vi "RunAClone.vi"(11 "VI in":refnum<vi>) -> (3 "reference out":refnum<vi>)   [LabVIEW 2021]
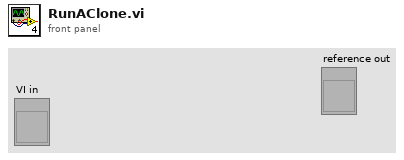
[diagram p1: front panel]
types:
  T1 = enum32{"Invalid", "Standard", "Closed", "Hidden", "Minimized", "Maximized"}
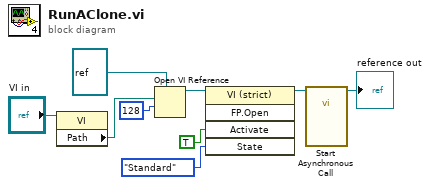
[diagram p0: block diagram]
diagram:
  n1 = property class="VI"(reference="VI in") -> ("Path"=w3:path)  [unwired: 1 in, 2 out]
  n2 = Open VI Reference(type specifier VI Refnum (for type only)=refnum<vi> refnum, vi path=w3, options=128) -> (vi reference=w8:refnum<vi>)  [unwired: 3 in, 1 out]
  n3 = invoke class="VI (strict)" method="FP.Open"(reference=w8, "Activate"=TRUE ("Activate?"), "State"=T1."Standard") -> (reference out=w9:refnum<vi>)  [unwired: 2 in, 4 out]
  n4 = call-by-ref "Start Asynchronous Call"(reference=w9) -> (reference out=→"reference out":refnum<vi>)  [unwired: 13 in, 1 out]
